vi "tsapp_clear_bus_statistics.vi"(8 "错误输入（无错误）":errorcluster) -> (0 "错误输出":errorcluster, 3 "tsapp_clear_bus_statistics":i32)   [LabVIEW 2016]
uses:
  TSMaster.dll
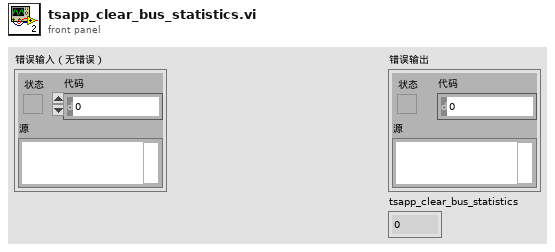
[diagram p1: front panel]
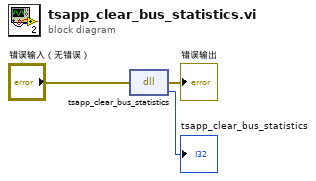
[diagram p0: block diagram]
diagram:
  n1 = dll-call lib="C:/Users/Eric/Desktop/LabVIEW/TSMasterAPI/Win32/CANopen_TS_2015/TSMaster.dll" fn="tsapp_clear_bus_statistics"(error in="错误输入（无错误）") -> (error out=→"错误输出":errorcluster, "tsapp_clear_bus_statistics"=→"tsapp_clear_bus_statistics":i32)  [unwired: 2 in, 1 out]
